vi "File Path.vi"(8 "error in (no error)":errorcluster, 10 "FileFullName":string, 11 "File FolderName":string(combo)="NULL") -> (0 "error out":errorcluster, 3 "File path":path)   [LabVIEW 2021]
uses:
  TopPath/TopPath.lvlib
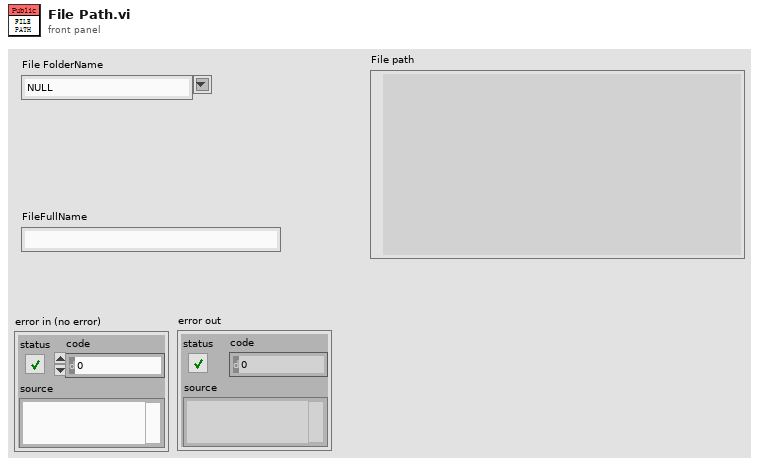
[diagram p1: front panel]
types:
  T1 = typedef "TopPath.lvlib/Top Path.ctl" = cluster{"LV Source":path, "FilePath":path, "Data":path}
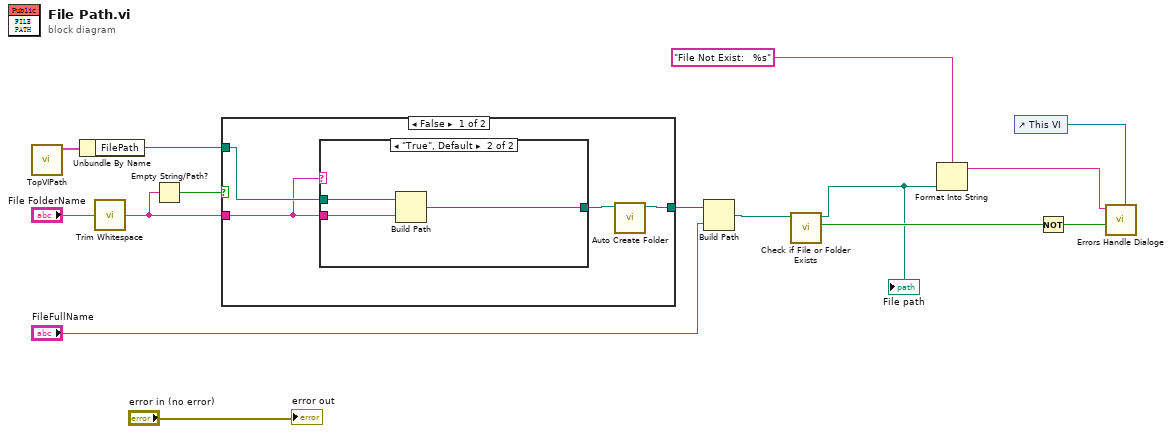
[diagram p0: block diagram]
diagram:
  n1 = call "TopVIPath.vi"() -> ("TopPath"=w15:T1)  [unwired: 10 in, 1 out]
  n2 = Unbundle By Name(w15) -> ("FilePath"=w14:path)
  n3 = call <vilib>:"Trim Whitespace.vi"("string"="File FolderName") -> ("trimmed string"=w9:string)  [unwired: 1 in]
  n4 = Empty String/Path?(string/path=w9) -> (empty?=w8:bool)
  n5 = case shown="False" w8 {
    tunnel: w14 -> [w19 w24]
    tunnel: [w16 w24] -> w13
    tunnel: w9 -> [w18 _]
    frame False {
      n6 = case shown="\"True\", Default" w18 {
        tunnel: w19 -> [w20 w23]
        tunnel: [w20 w22] -> w17
        tunnel: w18 -> [_ w21]
        frame "NULL" {
        }
        frame "True", Default {
          n7 = Build Path(base path=w23, name or relative path=w21) -> (appended path=w22:path)
        }
      }
      n8 = call "Auto Create Folder.vi"("Folder path"=w17) -> ("Folder path"=w16:path)  [unwired: 9 in, 1 out]
    }
    frame True {
    }
  }
  n9 = Build Path(base path=w13, name or relative path="FileFullName") -> (appended path=w7:path)
  n10 = call <vilib>:"Check if File or Folder Exists.vi"("path"=w7) -> ("file or folder exists?"=w6:bool, "dup path"=w3:path)  [unwired: 8 in, 1 out]
  "File path" <- w3
  n11 = Format Into String(format string="File Not Exist:   %s", w3) -> (resulting string=w2:string)  [unwired: 2 in, 1 out]
  n12 = control-ref of="This VI"() -> (w1:refnum<vi>)
  n13 = Not(x=w6) -> (.not. x?=w5:bool)
  n14 = call <userlib>:"Errors Handle Dialoge.vi"("VI Ref"=w1, "DisplayDialog"=w5, "Message"=w2) -> ()  [unwired: 7 in, 2 out]
  "error out" <- "error in (no error)"
